vi "Send_Configuration_Zurich.vi"(2 "Filename (.ini)":string="Config_Ver_1\\Zurich_params.ini", 3 "Handle In":T1 {"Handle" format="0x%08x"; "Conn" format="0x%08x"}, 4 "ModHandle In":T2 {"ModHandle" format="0x%08x"; "Conn" format="0x%08x"}, 7 "error in":errorcluster) -> (0 "Handle Out":T1 {"Handle" format="0x%08x"; "Conn" format="0x%08x"}, 1 "ModHandle Out":T2 {"ModHandle" format="0x%08x"; "Conn" format="0x%08x"}, 5 "error out":errorcluster)   [LabVIEW 2021]
uses:
  <instrlib>/Zurich Instruments LabOne/Public/Modules/ziTypeModHandle.ctl
  <instrlib>/Zurich Instruments LabOne/Public/ziTypeHandle.ctl
  <instrlib>/Zurich Instruments LabOne/Public/Modules/ziModSetValueBinaryArray.vi
  <instrlib>/Zurich Instruments LabOne/Public/Modules/ziModSetValueDoubleArray.vi
  <instrlib>/Zurich Instruments LabOne/Public/Configure/ziSetValueDouble.vi
  <instrlib>/Zurich Instruments LabOne/Public/Configure/ziSetValueBinary.vi
  <instrlib>/Zurich Instruments LabOne/Zurich Instruments LabOne.lvlib
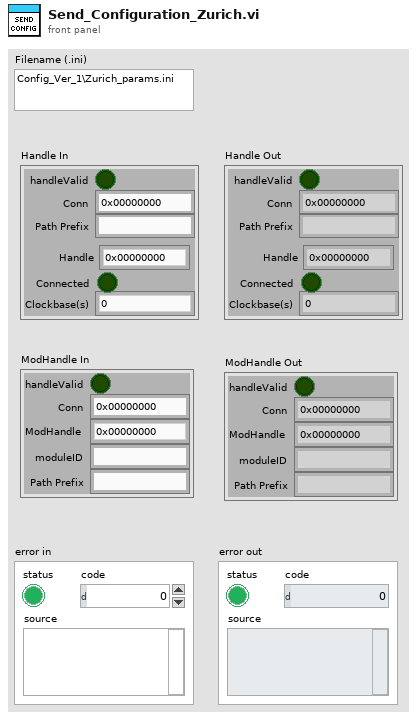
[diagram p1: front panel]
types:
  T1 = typedef "Zurich Instruments LabOne.lvlib/ziTypeHandle.ctl" = cluster{"handleValid":bool, "Conn":u64, "Path Prefix":string, "Handle":u64, "Clockbase(s)":dbl, "Connected":bool}
  T2 = typedef "Zurich Instruments LabOne.lvlib/ziTypeModHandle.ctl" = cluster{"handleValid":bool, "Conn":u64, "ModHandle":u64, "moduleID":string, "Path Prefix":string}
  T3 = cluster{"command":string[], "value":string[], "section exist(?)":bool}
  T4 = cluster{"command":string[], "value":dbl[], "section exist(?)":bool}
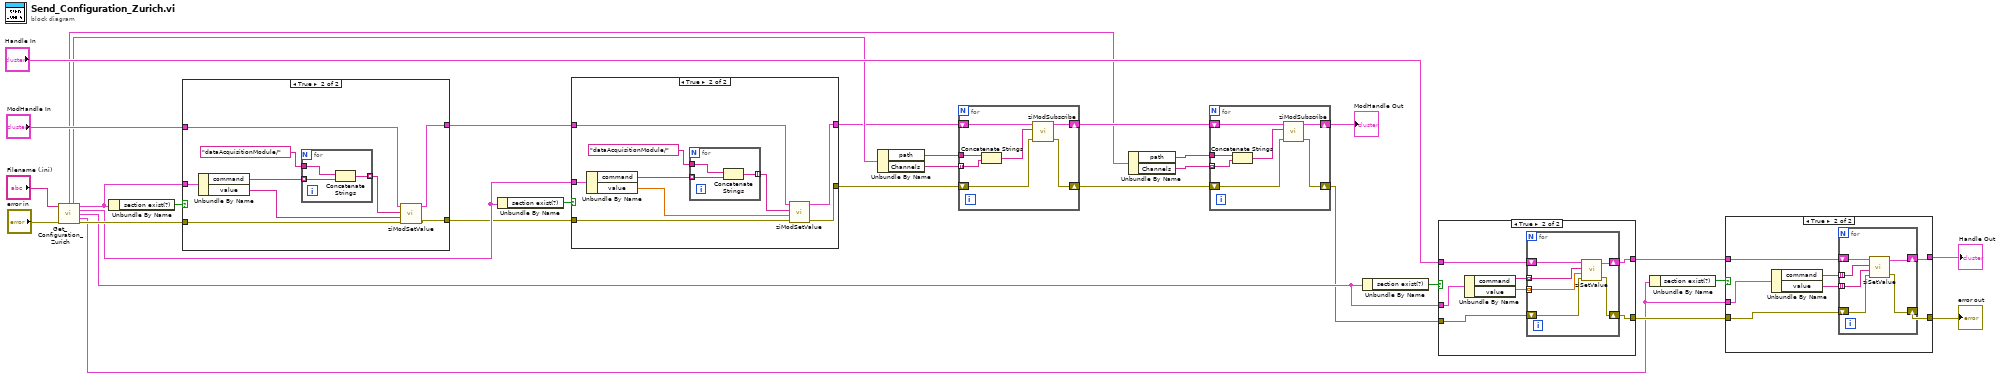
[diagram p0: block diagram]
diagram:
  n1 = call "Get_Configuration_Zurich.vi"("Filename (.ini)"="Filename (.ini)", "error in"="error in") -> ("Subscription 3"=w1:cluster{"path":string, "Channels":string[]}, "Subscription 0"=w12:cluster{"path":string, "Channels":string[]}, "data Acquisition Module string"=w29:T3, "data Acquisition Module double"=w25:T4, "general settings double"=w20:T4, "general settings string"=w16:T3, "error out"=w28:errorcluster)  [unwired: 7 in]
  n2 = Unbundle By Name(w29) -> ("section exist(?)"=w30:bool)
  n3 = case shown="True" w30 {
    tunnel: w29 -> [_ w42]
    tunnel: w28 -> [w32 w37]
    tunnel: "ModHandle In" -> [w33 w36]
    tunnel: [w32 w35] -> w24
    tunnel: [w33 w34] -> w23
    frame False {
    }
    frame True {
      n4 = Unbundle By Name(w42) -> ("command"=w41:string[], "value"=w38:string[])
      n5 = for {
        tunnel: w41 -> [w44] mode=indexing
        tunnel: "dataAcquisitionModule/" -> [w45]
        tunnel: [w43] -> w39 mode=indexing
        n6 = Concatenate Strings(w45, w44) -> (w43:string)
      }
      n7 = call-poly <instrlib>:"ziModSetValue.vi"("Error In"=w37, "Values"=w38, "Paths"=w39, "ModHandle In"=w36) -> ("Error Out"=w35:errorcluster, "ModHandle Out"=w34:T2)  [unwired: 6 in]
    }
  }
  n8 = Unbundle By Name(w25) -> ("section exist(?)"=w26:bool)
  n9 = case shown="True" w26 {
    tunnel: w25 -> [_ w56]
    tunnel: w24 -> [w46 w51]
    tunnel: w23 -> [w47 w50]
    tunnel: [w47 w49] -> w9
    tunnel: [w46 w48] -> w8
    frame False {
    }
    frame True {
      n10 = Unbundle By Name(w56) -> ("command"=w55:string[], "value"=w52:dbl[])
      n11 = for {
        tunnel: w55 -> [w58] mode=indexing
        tunnel: "dataAcquisitionModule/" -> [w59]
        tunnel: [w57] -> w53 mode=indexing
        n12 = Concatenate Strings(w59, w58) -> (w57:string)
      }
      n13 = call-poly <instrlib>:"ziModSetValue.vi"("Error In"=w51, "Values"=w52, "Paths"=w53, "ModHandle In"=w50) -> ("Error Out"=w48:errorcluster, "ModHandle Out"=w49:T2)  [unwired: 6 in]
    }
  }
  n14 = Unbundle By Name(w12) -> ("path"=w11:string, "Channels"=w10:string[])
  n15 = for {
    tunnel: w11 -> [w64]
    tunnel: w10 -> [w63] mode=indexing
    shift-right: [w65] -> w4
    shift-left: w9 -> [w66]
    shift-right: [w60] -> w3
    shift-left: w8 -> [w61]
    n16 = Concatenate Strings(w64, w63) -> (w62:string)
    n17 = call <instrlib>:"ziModSubscribe.vi"("Error In"=w61, "Path"=w62, "ModHandle In"=w66) -> ("Error Out"=w60:errorcluster, "ModHandle Out"=w65:T2)  [unwired: 6 in]
  }
  n18 = Unbundle By Name(w1) -> ("path"=w6:string, "Channels"=w7:string[])
  n19 = for {
    tunnel: w6 -> [w71]
    tunnel: w7 -> [w70] mode=indexing
    shift-right: [w72] -> w5
    shift-left: w4 -> [w73]
    shift-right: [w67] -> w2
    shift-left: w3 -> [w68]
    n20 = Concatenate Strings(w71, w70) -> (w69:string)
    n21 = call <instrlib>:"ziModSubscribe.vi"("Error In"=w68, "Path"=w69, "ModHandle In"=w73) -> ("Error Out"=w67:errorcluster, "ModHandle Out"=w72:T2)  [unwired: 6 in]
  }
  "ModHandle Out" <- w5
  n22 = Unbundle By Name(w20) -> ("section exist(?)"=w21:bool)
  n23 = case shown="True" w21 {
    tunnel: "Handle In" -> [w75 w82]
    tunnel: w2 -> [w74 w81]
    tunnel: w20 -> [_ w76]
    tunnel: [w74 w80] -> w18
    tunnel: [w75 w79] -> w17
    frame False {
    }
    frame True {
      n24 = Unbundle By Name(w76) -> ("command"=w78:string[], "value"=w77:dbl[])
      n25 = for {
        shift-right: [w87] -> w79
        shift-left: w82 -> [w88]
        shift-right: [w85] -> w80
        shift-left: w81 -> [w86]
        tunnel: w78 -> [w84] mode=indexing
        tunnel: w77 -> [w83] mode=indexing
        n26 = call-poly <instrlib>:"ziSetValue.vi"("Error In"=w86, "Value"=w83, "Path"=w84, "Handle In"=w88) -> ("Error Out"=w85:errorcluster, "Handle Out"=w87:T1)  [unwired: 1 in]
      }
    }
  }
  n27 = Unbundle By Name(w16) -> ("section exist(?)"=w19:bool)
  n28 = case shown="True" w19 {
    tunnel: w17 -> [w90 w97]
    tunnel: w18 -> [w89 w96]
    tunnel: w16 -> [_ w93]
    tunnel: [w90 w95] -> w15
    tunnel: [w89 w94] -> w13
    frame False {
    }
    frame True {
      n29 = Unbundle By Name(w93) -> ("command"=w92:string[], "value"=w91:string[])
      n30 = for {
        shift-right: [w100] -> w95
        shift-left: w97 -> [w103]
        shift-right: [w101] -> w94
        shift-left: w96 -> [w102]
        tunnel: w92 -> [w99] mode=indexing
        tunnel: w91 -> [w98] mode=indexing
        n31 = call-poly <instrlib>:"ziSetValue.vi"("Error In"=w102, "Data"=w98, "Path"=w99, "Handle In"=w103) -> ("Error Out"=w101:errorcluster, "Handle Out"=w100:T1)  [unwired: 1 in]
      }
    }
  }
  "Handle Out" <- w15
  "error out" <- w13
